vi "organizeBufferToVolumeForDisplay.vi"(10 "buffer":u32[](array[numeric]), 11 "volume info":T1) -> (1 "fb only (image if no ff/fb)":u32[][][](array[numeric]), 2 "ff only (0 if no ff/fb)":u32[][][](array[numeric]), 3 "image":u32[][][](array[numeric]))   [LabVIEW 2010]
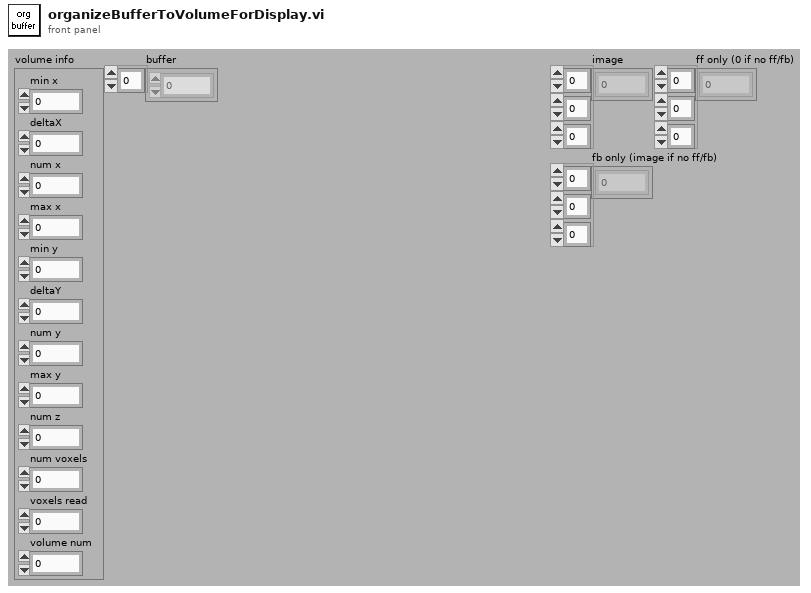
[diagram p1: front panel]
types:
  T1 = cluster{"min x":i16, "deltaX":dbl, "num x":u32, "max x":i16, "min y":i16, "deltaY":dbl, "num y":u32, "max y":i16, "num z":u32, "num voxels":u32, "voxels read":u32, "volume num":u32}
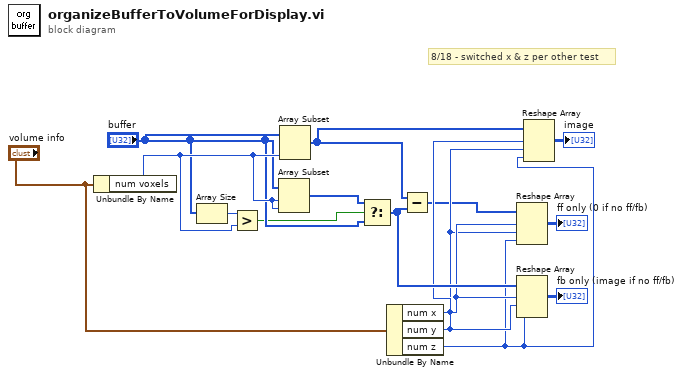
[diagram p0: block diagram]
diagram:
  # "8/18 - switched x & z per other test"
  n1 = Unbundle By Name("volume info") -> ("num voxels"=w14:u32)
  n2 = Array Size(array="buffer") -> (size(s)=w15:i32)
  n3 = Greater?(x=w15, y=w14) -> (0:w11:bool)
  n4 = Array Subset(array="buffer", index=w14, length=w14) -> (w13:u32[])
  n5 = Array Subset(array="buffer", length=w14) -> (w10:u32[])  [unwired: 1 in]
  n6 = Select(t=w13, s=w11, f="buffer") -> (s? t:f=w9:u32[])
  n7 = Unbundle By Name("volume info") -> ("num x"=w7:u32, "num y"=w6:u32, "num z"=w5:u32)
  n8 = Subtract(x=w10, y=w9) -> (x-y=w1:u32[])
  n9 = Reshape Array(w1, w7, w6, w5) -> (→"ff only (0 if no ff/fb)":u32[][][])
  n10 = Reshape Array(w9, w7, w6, w5) -> (→"fb only (image if no ff/fb)":u32[][][])
  n11 = Reshape Array(w10, w7, w6, w5) -> (→"image":u32[][][])
